vi "归零时间.vi"(3 "计算参数 in":T2, 4 "输入参数 in":T1, 5 "进油口压力":dbl[](array[numeric]), 6 "Array in":dbl[](array[numeric])) -> (0 "计算参数 out":T2, 2 "Waveform Graph":cluster{dbl, dbl, dbl[][]}(graph))   [LabVIEW 2013]
doc: "此程序计算归零时间\nDFT=td1-td"
panel:
  out "Array out":dbl[](array[numeric])
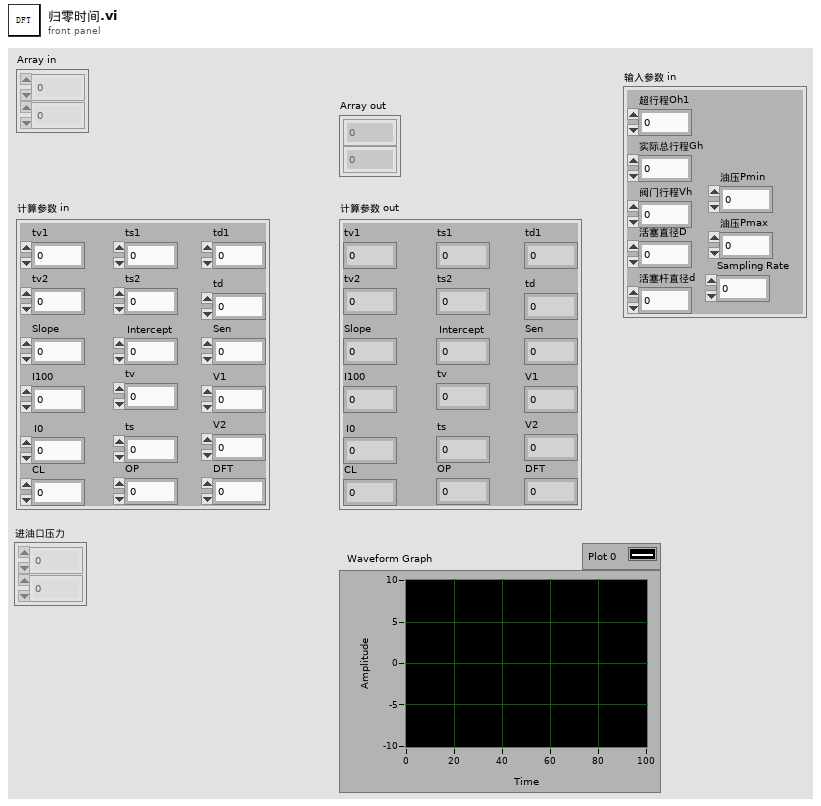
[diagram p1: front panel]
types:
  T1 = cluster{"超行程Oh1":dbl, "实际总行程Gh":dbl, "阀门行程Vh":dbl, "活塞直径D":dbl, "活塞杆直径d":dbl, "油压Pmin":dbl, "油压Pmax":dbl, "Sampling Rate":dbl}
  T2 = cluster{"tv1":dbl, "tv2":dbl, "tv":dbl, "ts1":dbl, "ts2":dbl, "ts":dbl, "td1":dbl, "td":dbl, "Slope":dbl, "Intercept":dbl, "I100":dbl, "I0":dbl, "Sen":dbl, "V1":dbl, "V2":dbl, "CL":dbl, "OP":dbl, "DFT":dbl}
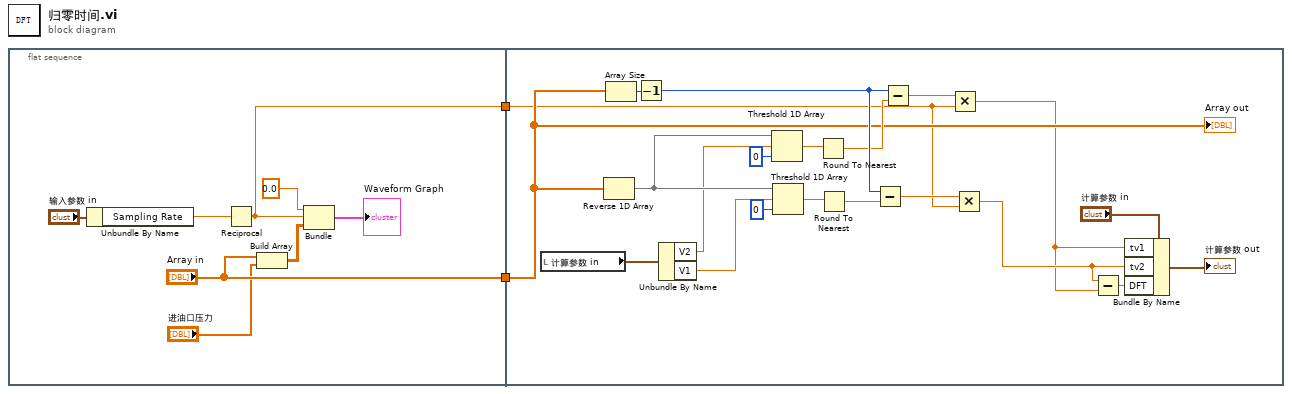
[diagram p0: block diagram]
diagram:
  n1 = flat-sequence {
    tunnel: ["Array in"] -> w2
    tunnel: [w8] -> w1
    tunnel: w2 -> [w16]
    tunnel: w1 -> [w13]
    frame #0 {
      n2 = Unbundle By Name("输入参数 in") -> ("Sampling Rate"=w3:dbl)
      n3 = Reciprocal(x=w3) -> (1/x=w8:dbl)
      n4 = Build Array("Array in", "进油口压力") -> (w5:dbl[][])
      n5 = Bundle(0.0, w8, w5) -> (→"Waveform Graph":cluster{dbl, dbl, dbl[][]})  [unwired: 1 in]
    }
    frame #1 {
      n6 = local read "计算参数 in"() -> (w19:T2)
      n7 = Reverse 1D Array(array=w16) -> (reversed array=w27:dbl[])
      n8 = Array Size(array=w16) -> (size(s)=w28:i32)
      n9 = Decrement(x=w28) -> (x-1=w30:i32)
      n10 = Unbundle By Name(w19) -> ("V2"=w26:dbl, "V1"=w25:dbl)
      n11 = Threshold 1D Array(1:0 ("start index (0)"), 2:w26, 3:w27) -> (0:w20:dbl)
      n12 = Threshold 1D Array(1:0 ("start index (0)"), 2:w25, 3:w27) -> (0:w21:dbl)
      n13 = Round To Nearest(number=w20) -> (nearest integer value=w29:dbl)
      n14 = Round To Nearest(number=w21) -> (nearest integer value=w31:dbl)
      n15 = Subtract(x=w30, y=w31) -> (x-y=w14:dbl)
      n16 = Subtract(x=w30, y=w29) -> (x-y=w15:dbl)
      n17 = Multiply(x=w15, y=w13) -> (x*y=w11:dbl)
      n18 = Multiply(x=w14, y=w13) -> (x*y=w12:dbl)
      n19 = Subtract(x=w12, y=w11) -> (x-y=w24:dbl)
      n20 = Bundle By Name(cluster="计算参数 in", "tv1"=w11, "tv2"=w12, "DFT"=w24) -> (→"计算参数 out":T2)
      "Array out" <- w16
    }
  }
